vi "GetCtrlsRefByName_ArrGen.vi"(7 "Commandes []":refnum<vi>[](array[refnum]), 8 "ErrorIn(No Error)":errorcluster caption="entrée d'erreur (pas d'erreur)", 9 "ControlName":string[](array[string]), 10 "InclTabCTrl":bool, 11 "VIRef":refnum<vi>) -> (0 "sortie d'erreur":errorcluster, 1 "Index":i32[](array[numeric]), 2 "ControlsRefs":refnum<vi>[](array[refnum]), 3 "AllControlsNames":string[](array[string]))   [LabVIEW 2019]
uses:
  Programmes Labview/LabScanV1A/DevicesClass/InstrumentsClass/DAQ6363/DAQ6363.lvclass
  <vilib>/Utility/error.llb/Error Cluster From Error Code.vi
  <vilib>/ErrorRing/Error Ring.xnode
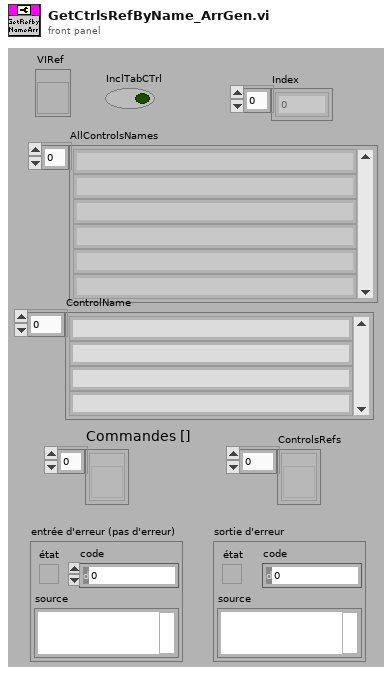
[diagram p1: front panel]
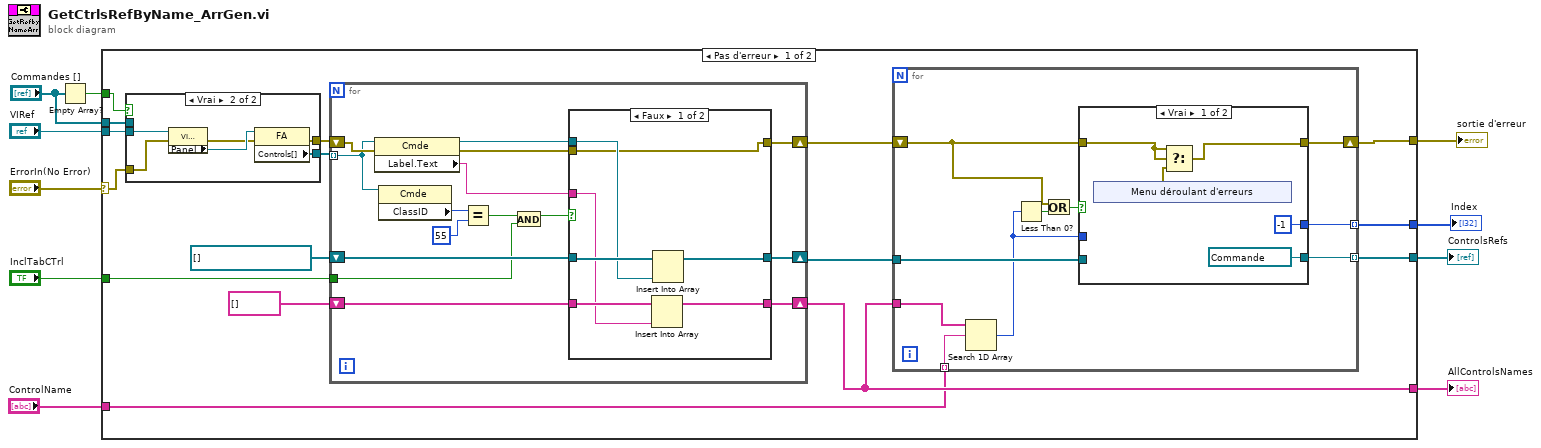
[diagram p0: block diagram]
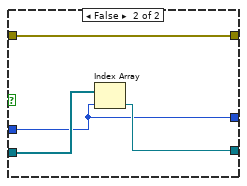
[diagram p2: hidden frame]
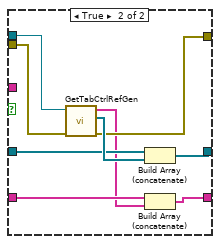
[diagram p4: hidden frame]
diagram:
  n1 = Empty Array?(array="Commandes []") -> (empty?=w3:bool)
  n2 = case shown="Pas d'erreur" "ErrorIn(No Error)" {
    selector: "ErrorIn(No Error)" -> [w24 w90]
    tunnel: [w17 w90] -> w9
    tunnel: "VIRef" -> [w26 _]
    tunnel: [w19 _] -> w7
    tunnel: "InclTabCTrl" -> [w22 _]
    tunnel: "ControlName" -> [w18 _]
    tunnel: [w15 _] -> w4
    tunnel: w3 -> [w12 _]
    tunnel: "Commandes []" -> [w13 _]
    tunnel: [w11 _] -> w1
    frame No Error {
      n3 = case shown="Vrai" w12 {
        tunnel: w26 -> [_ w56]
        tunnel: [w52 w55] -> w25
        tunnel: w24 -> [w51 w53]
        tunnel: [w51 w54] -> w23
        tunnel: w13 -> [w52 _]
        frame False {
        }
        frame True {
          n4 = property class="VI (strict)"(reference=w56, error in=w53) -> (error out=w57:errorcluster, "Panel"=w58:refnum<vi>)  [unwired: 1 out]
          n5 = property class="FA"(reference=w58, error in=w57) -> (error out=w54:errorcluster, "Controls[]"=w55:refnum<vi>[])  [unwired: 1 out]
        }
      }
      n6 = for {
        tunnel: w25 -> [w72] mode=indexing
        shift-right: [w61] -> w14
        shift-left: w23 -> [w73]
        shift-right: [w66] -> w16
        shift-left: refnum<vi>[] [] -> [w65]
        shift-right: [w64] -> w19
        shift-left: string[] [] -> [w62]
        tunnel: w22 -> [w60]
        n7 = property class="Cmde"(reference=w72, error in=w73) -> (reference out=w68:refnum<vi>, error out=w63:errorcluster, "Label.Text"=w69:string)
        n8 = property class="Cmde"(reference=w72) -> ("ClassID"=w71:u32)  [unwired: 1 in, 2 out]
        n9 = Equal?(x=w71, y=u32 55) -> (x = y?=w67:bool)
        n10 = And(x=w67, y=w60) -> (x .and. y?=w59:bool)
        n11 = case shown="Faux" w59 {
          tunnel: w69 -> [w76 _]
          tunnel: w68 -> [w75 w89]
          tunnel: [w80 w86] -> w66
          tunnel: w65 -> [w79 w84]
          tunnel: [w78 w87] -> w64
          tunnel: w63 -> [w74 w83]
          tunnel: w62 -> [w77 w88]
          tunnel: [w74 w82] -> w61
          frame False {
            n12 = Insert Into Array(array=w77, new element=w76) -> (w78:string[])  [unwired: 1 in]
            n13 = Insert Into Array(array=w79, new element=w75) -> (w80:refnum<vi>[])  [unwired: 1 in]
          }
          frame True {
            n14 = call <userlib>:"GetTabCtrlRefGen.vi"("ErrorIn(No Error)"=w83, "CommandRef"=w89) -> ("sortie d'erreur"=w82:errorcluster, "ControlsRefs"=w85:refnum<vi>[], "ControlsNames"=w81:string[])  [unwired: 7 in]
            n15 = Build Array (concatenate)(w84, w85) -> (w86:refnum<vi>[])
            n16 = Build Array (concatenate)(w88, w81) -> (w87:string[])
          }
        }
      }
      n17 = for {
        tunnel: w19 -> [w36]
        tunnel: w18 -> [w35] mode=indexing
        tunnel: w16 -> [w33]
        tunnel: [w32] -> w15 mode=indexing
        shift-right: [w34] -> w17
        shift-left: w14 -> [w29]
        tunnel: [w27] -> w11 mode=indexing
        n18 = Search 1D Array(1D array=w36, element=w35) -> (index of element=w28:i32)  [unwired: 1 in]
        n19 = Less Than 0?(x=w28) -> (x < 0?=w30:bool)
        n20 = Or(x=w29, y=w30) -> (x .or. y?=w31:bool)
        n21 = case shown="Vrai" w31 {
          tunnel: [w40 w50] -> w34
          tunnel: w29 -> [w41 w50]
          tunnel: w33 -> [_ w49]
          tunnel: [refnum<vi> refnum ("CommandRef") w48] -> w32
          tunnel: w28 -> [_ w47]
          tunnel: [-1 ("index of element") w47] -> w27
          frame True {
            n22 = xnode "Menu déroulant d'erreurs"() -> ("sortie d'erreur"=w39:errorcluster)
            n23 = Select(t=w41, s=w41, f=w39) -> (s? t:f=w40:errorcluster)
          }
          frame False {
            n24 = Index Array(array=w49, index=w47) -> (element=w48:refnum<vi>)
          }
        }
      }
    }
    frame Error {
    }
  }
  "sortie d'erreur" <- w9
  "AllControlsNames" <- w7
  "ControlsRefs" <- w4
  "Index" <- w1
